vi "Identities.vi"(8 "error in (no error)":errorcluster, 11 "DataLoggerAPI in":refnum<class "DataLoggerAPI.lvclass">) -> (0 "error out":errorcluster, 2 "Identities":refnum<class "Identity.lvclass">[](array[class]), 3 "DataLoggerAPI out":refnum<class "DataLoggerAPI.lvclass">)   [LabVIEW 2020, in "VolatusDataLogger.lvlib" / "DataLoggerAPI.lvclass"]
uses:
  DataLoggerAPI.lvclass
  Volatus/Identity/Identity.lvclass
  DataLoggerAPI.lvclass/DataLoggerAPI.ctl
  DataLoggerIdentity/DataLoggerIdentity.lvclass
  C:/dev/lv20CE/relink/lv-volatus/Volatus/Identity/Identity.lvclass
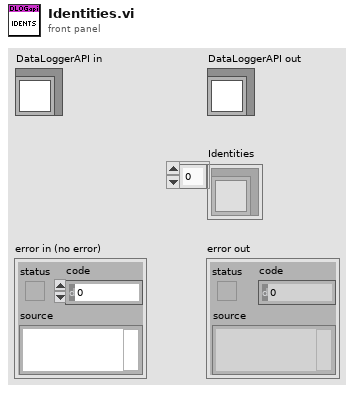
[diagram p1: front panel]
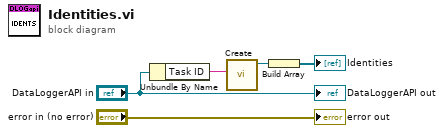
[diagram p0: block diagram]
diagram:
  n1 = Unbundle By Name("DataLoggerAPI in") -> ("Task ID"=w3:string)
  n2 = call "Create.vi"("Task ID"=w3) -> ("DataLoggerIdentity out"=w2:refnum<class "DataLoggerIdentity.lvclass">)  [unwired: 10 in]
  n3 = Build Array(w2) -> (→"Identities":refnum<class "DataLoggerIdentity.lvclass">[])
  "error out" <- "error in (no error)"
  "DataLoggerAPI out" <- "DataLoggerAPI in"
